vi "MediaAdapter.vi"(8 "error in (no error)":errorcluster, 10 "audioType":string, 11 "MediaAdapter in":refnum<class "MediaAdapter.lvclass">) -> (0 "error out":errorcluster, 3 "MediaAdapter out":refnum<class "MediaAdapter.lvclass">)   [LabVIEW 2017, in "MediaAdapter.lvclass"]
uses:
  MediaAdapter.lvclass
  Mp4Player/Mp4Player.lvclass
  C:/Users/fflores/Documents/LabVIEW-Open-Projects/LabIVEW OOP Design Patterns/Adapter Pattern/Media Player Example/Advanced Media Player/AdvancedMediaPlayer.lvclass
  MediaAdapter.lvclass/MediaAdapter.ctl
  VlcPlayer/VlcPlayer.lvclass
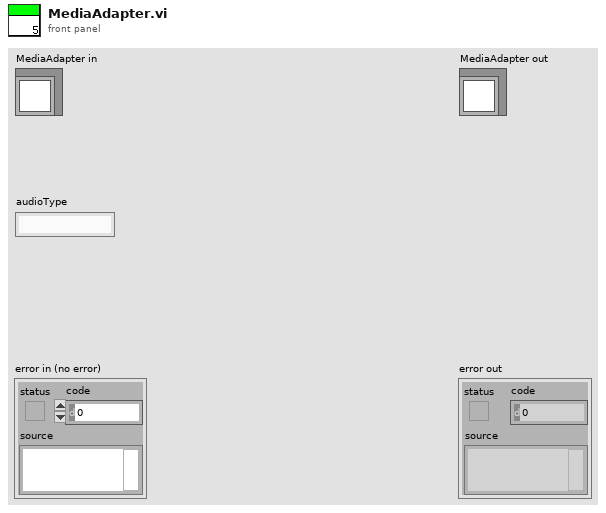
[diagram p1: front panel]
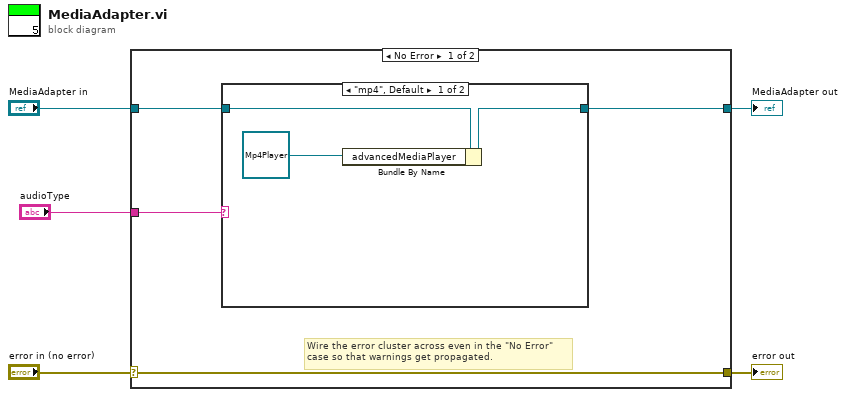
[diagram p0: block diagram]
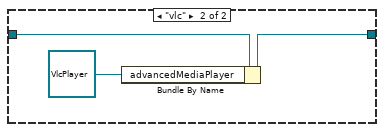
[diagram p2: hidden frame]
diagram:
  n1 = case shown="No Error" "error in (no error)" {
    selector: "error in (no error)" -> [w9 w17]
    tunnel: [w9 w17] -> w4
    tunnel: [w7 w16] -> w2
    tunnel: "MediaAdapter in" -> [w6 w16]
    tunnel: "audioType" -> [w8 _]
    frame No Error {
      # "Wire the error cluster across even in the \"No Error\"\ncase so that warnings get propagated."
      n2 = case shown="\"mp4\", Default" w8 {
        tunnel: [w11 w14] -> w7
        tunnel: w6 -> [w12 w15]
        frame "mp4", Default {
          n3 = Bundle By Name(cluster=w12, "advancedMediaPlayer"=refnum<class "Mp4Player.lvclass"> refnum ("Mp4Player.lvclass")) -> (w11:refnum<class "MediaAdapter.lvclass">)
        }
        frame "vlc" {
          n4 = Bundle By Name(cluster=w15, "advancedMediaPlayer"=refnum<class "VlcPlayer.lvclass"> refnum ("VlcPlayer.lvclass")) -> (w14:refnum<class "MediaAdapter.lvclass">)
        }
      }
    }
    frame Error {
    }
  }
  "error out" <- w4
  "MediaAdapter out" <- w2
